vi "MainMyRIO.vi"() -> ()   [LabVIEW 2016]
uses:
  <vilib>/myRIO/Instrument Drivers/Onboard Devices/Accelerometer/typedefs/Accelerometer Reference.ctl
  <vilib>/myRIO/Common/Instrument Driver Framework/Utilities/typedefs/myRIO Generic Hardware Reference.ctl
  <vilib>/myRIO/Common/Instrument Driver Framework/Utilities/typedefs/Hardware Version Enum.ctl
  <vilib>/myRIO/Common/Instrument Driver Framework/Utilities/typedefs/myRIO v1.0 Reference.ctl
  <vilib>/myRIO/Common/Instrument Driver Framework/Utilities/typedefs/Generic FPGA Reference.ctl
  <vilib>/myRIO/Common/Instrument Driver Framework/myRIO v1.0/Accelerometer/typedefs/Accelerometer Channels List.ctl
  <vilib>/myRIO/Common/Instrument Driver Framework/myRIO v1.0/Accelerometer/typedefs/Accelerometer Channels Enum.ctl
  <vilib>/userdefined/High Color/nirio_resource_hc.ctl
  Data.ctl
  <vilib>/myRIO/Common/Instrument Driver Framework/myRIO v1.0/Accelerometer/vis/myRIO v1.1 Open Accelerometer.vi
  <vilib>/myRIO/Common/Instrument Driver Framework/Utilities/vis/Validate Channels.vi
  <vilib>/myRIO/Common/Instrument Driver Framework/myRIO v1.0/Accelerometer/vis/myRIO v1.0 Reserve Accelerometer.vi
  <vilib>/myRIO/Common/Instrument Driver Framework/myRIO v1.0/Accelerometer/vis/myRIO v1.0 Close Accelerometer.vi
  <vilib>/myRIO/Common/Instrument Driver Framework/myRIO v1.0/Resource Manager/vis/myRIO v1.0 Reserve Channel List.vi
  <vilib>/myRIO/Common/Instrument Driver Framework/myRIO v1.0/Accelerometer/vis/myRIO v1.0 Build MUX Configuration Accelerometer.vi
  <vilib>/myRIO/Common/Instrument Driver Framework/myRIO v1.0/Accelerometer/vis/myRIO v1.0 Unreserve Accelerometer.vi
  <vilib>/myRIO/Common/Instrument Driver Framework/myRIO v1.0/Resource Manager/vis/myRIO v1.0 Reserve Channel.vi
  <vilib>/myRIO/Common/Instrument Driver Framework/myRIO v1.0/Resource Manager/vis/myRIO v1.0 Unreserve Channel.vi
  <vilib>/myRIO/Common/Instrument Driver Framework/myRIO v1.0/Resource Manager/vis/myRIO v1.0 Unreserve Channel List.vi
  <vilib>/myRIO/Common/Instrument Driver Framework/myRIO v1.0/Resource Manager/vis/myRIO v1.0 Build Mutex Name.vi
  <vilib>/Utility/VariantDataType/GetNumericInfo.vi
  <vilib>/Utility/error.llb/Error Cluster From Error Code.vi
  <vilib>/myRIO/Common/Instrument Driver Framework/myRIO v1.0/myRIO v1.1 Open.vi
  <vilib>/myRIO/Common/Instrument Driver Framework/myRIO v1.0/Accelerometer/vis/myRIO v1.0 Get Scaling Constant Accelerometer.vi
  <vilib>/myRIO/Common/Instrument Driver Framework/Utilities/vis/IO Manager.vi
  <vilib>/myRIO/Common/Instrument Driver Framework/Utilities/vis/Configuration Manager.vi
  <vilib>/myRIO/Common/Instrument Driver Framework/myRIO v1.0/myRIO v1.0 Close.vi
  <vilib>/myRIO/Common/Instrument Driver Framework/myRIO v1.0/Accelerometer/vis/myRIO v1.0 Read Accelerometer.vi
  <vilib>/myRIO/Instrument Drivers/Onboard Devices/Accelerometer/vis/myRIO Accelerometer Open.xnode
  <vilib>/myRIO/Instrument Drivers/Onboard Devices/Accelerometer/Accelerometer.lvlib
panel:
  out "Iteration":i32
  out "Waveform Chart":T1(graph)
  in  "stop":bool
  in  "Start":bool
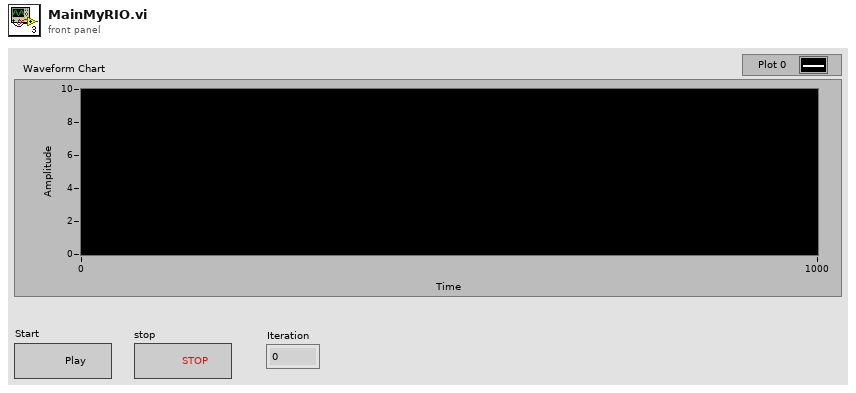
[diagram p1: front panel]
types:
  T1 = cluster{"Values[0]":dbl, "Values[1]":dbl, "Values[2]":dbl}
  T2 = typedef "Accelerometer.lvlib/Accelerometer Reference.ctl" = cluster{"myRIO Reference":T3, "Accelerometer Channels List":T7, "LSB Weight":dbl}
  T3 = typedef "myRIO Generic Hardware Reference.ctl" = cluster{"myRIO Model":T4, "myRIO Hardware Reference":T5}
  T4 = typedef "Hardware Version Enum.ctl" = enum16{"Unknown", "myRIO-1900", "myRIO-1950", "roboRIO", "NI ELVIS RIO CM"}
  T5 = typedef "myRIO v1.0 Reference.ctl" = cluster{"Generic FPGA Reference":T6, "Allow multiple opens":bool}
  T6 = typedef "Generic FPGA Reference.ctl" = refnum<k20>
  T7 = typedef "Accelerometer Channels List.ctl" = T8[]
  T8 = typedef "Accelerometer Channels Enum.ctl" = enum16{"Not Connected", "X-Axis", "Y-Axis", "Z-Axis"}
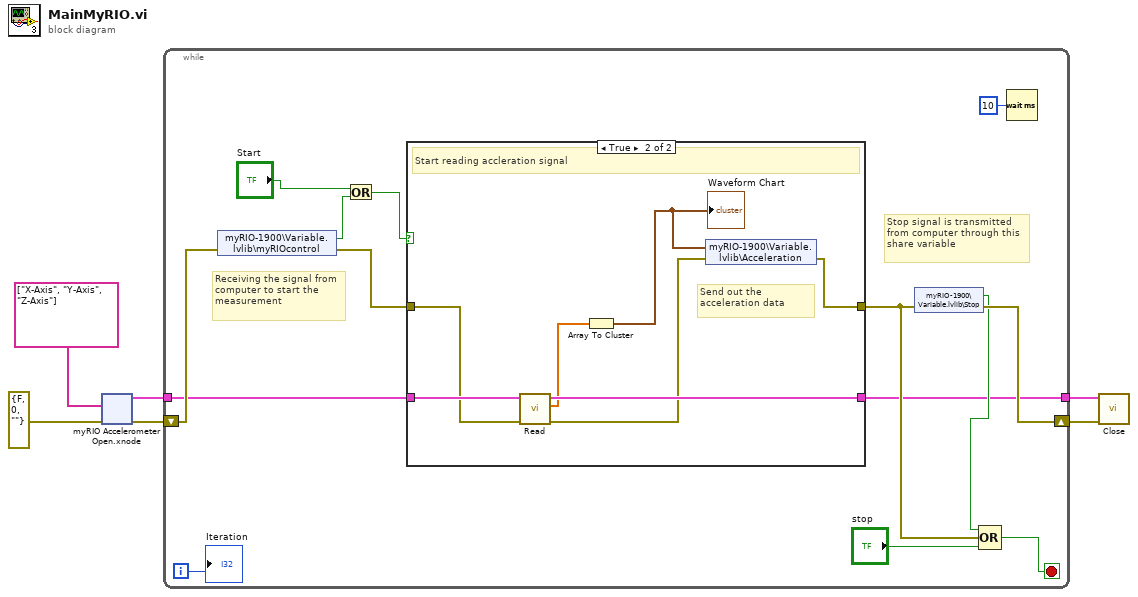
[diagram p0: block diagram]
diagram:
  n1 = xnode "myRIO Accelerometer Open.xnode"("error in (no error)"=errorcluster {"status"=FALSE, "code"=0, "source"=""} ("error IO"), "Channel Names"=tag[] ["X-Axis", "Y-Axis", "Z-Axis"]) -> ("error out"=w4:errorcluster, "Accelerometer Ref Out"=w6:T2)  [unwired: 1 in]
  n2 = while {
    shift-right: [w15] -> w3
    shift-left: w4 -> [w14]
    tunnel: w6 -> [w8]
    tunnel: [w7] -> w5
    i -> [w9]
    stop <- w13 stop-if-true
    # "Stop signal is transmitted from computer through this share variable"
    # "Receiving the signal from computer to start the measurement"
    n3 = shared-variable "myRIO-1900\\Variable.lvlib\\myRIOcontrol"(error in=w14) -> (w18:bool, error out=w19:errorcluster)
    n4 = Or(x="Start", y=w18) -> (x .or. y?=w16:bool)
    n5 = case shown="True" w16 {
      tunnel: w19 -> [w22 w24]
      tunnel: [w22 w29] -> w11
      tunnel: w8 -> [w21 w28]
      tunnel: [w21 w27] -> w7
      frame False {
        # "Do nothing"
      }
      frame True {
        # "Send out the acceleration data"
        # "Start reading accleration signal"
        n6 = call <vilib>:"Read.vi"("error in (no error)"=w24, "Accelerometer Ref In"=w28) -> ("error out"=w23:errorcluster, "Values"=w26:dbl[], "Accelerometer Ref Out"=w27:T2)  [unwired: 7 in]
        n7 = Array To Cluster(array=w26) -> (cluster=w25:T1)
        "Waveform Chart" <- w25
        n8 = shared-variable "myRIO-1900\\Variable.lvlib\\Acceleration"(w25, error in=w23) -> (error out=w29:errorcluster)
      }
    }
    n9 = shared-variable "myRIO-1900\\Variable.lvlib\\Stop"(error in=w11) -> (w10:bool, error out=w15:errorcluster)
    n10 = Compound Arithmetic op=OR(w10, w11, "stop") -> (w13:bool)
    n11 = Wait (ms)(milliseconds to wait=u32 10) -> ()  [unwired: 1 out]
    "Iteration" <- w9
  }
  n12 = call <vilib>:"Close.vi"("error in (no error)"=w3, "Accelerometer Ref In"=w5) -> ()  [unwired: 9 in, 1 out]
